vi "Turn to Angle.vi"(3 "PID Gains":T1 {"derivative time (Td, min)" format="%.3f"; "integral time (Ti, min)" format="%.3f"; "proportional gain (Kc)" format="%.3f"}, 4 "Rotation Multiplier":dbl, 5 "Target angle":dbl, 6 "Angle (radians; 0 = right)":dbl) -> (2 "Turn Set Point":dbl)   [LabVIEW 2015]
uses:
  <vilib>/addons/control/pid/pid.llb/PID Control Input Filter (DBL).vi
  <vilib>/addons/control/pid/pid.llb/PID (DBL).vi
  <vilib>/addons/control/pid/NI_PID_pid.lvlib
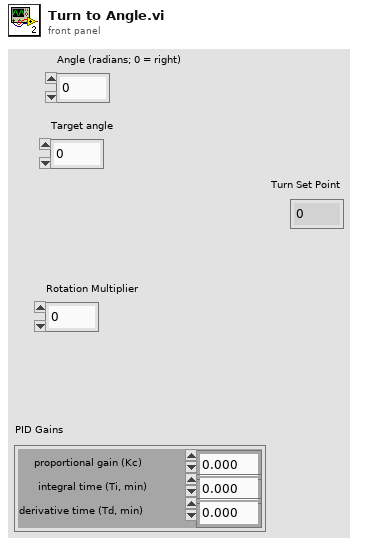
[diagram p1: front panel]
types:
  T1 = cluster{"proportional gain (Kc)":dbl, "integral time (Ti, min)":dbl, "derivative time (Td, min)":dbl}
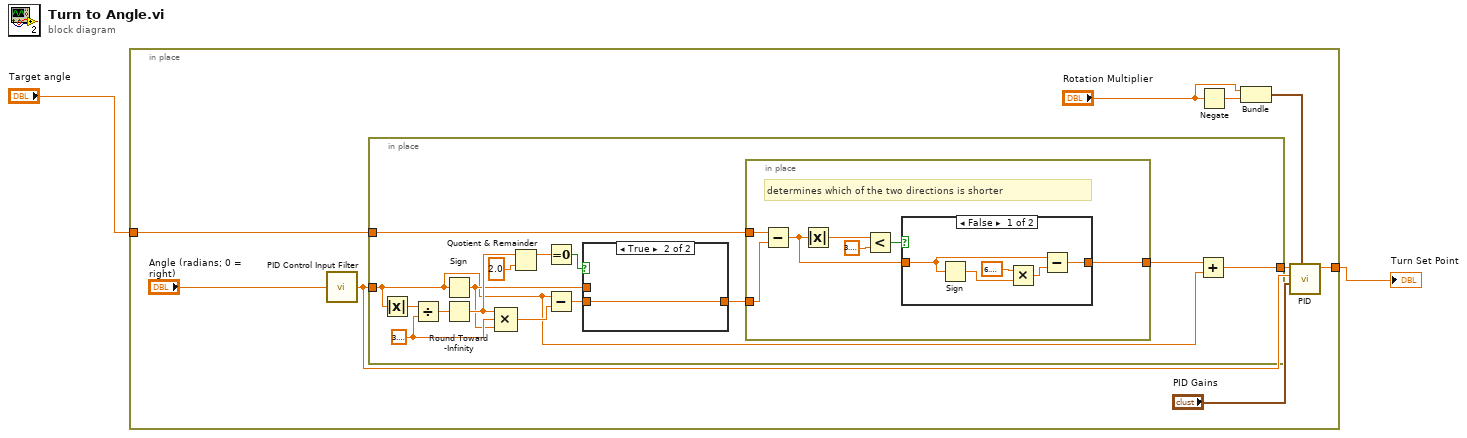
[diagram p0: block diagram]
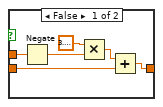
[diagram p3: hidden frame]
diagram:
  n1 = in-place {
    in-place-border: [w11] -> w1
    in-place-border: "Target angle" -> [w5]
    n2 = call-poly <vilib>:"PID Control Input Filter.vi"("input"="Angle (radians; 0 = right)") -> ("output"=w3:dbl)  [unwired: 4 in]
    n3 = in-place {
      in-place-border: w5 -> [w15]
      in-place-border: [w14] -> w4
      in-place-border: w3 -> [w12]
      w23 = 3.141592653589793
      n4 = Absolute Value(x=w12) -> (abs(x)=w26:dbl)
      n5 = Divide(x=w26, y=w23) -> (x/y=w25:dbl)
      n6 = Sign(1:w12) -> (0:w17:dbl)
      n7 = Round Toward -Infinity(1:w25) -> (0:w22:dbl)
      n8 = Compound Arithmetic op=MULTIPLY(w22, w23, w17) -> (w24:dbl)
      n9 = Quotient & Remainder(x=w22, y=2.0) -> (x-y*floor(x/y)=w20:dbl)  [unwired: 1 out]
      n10 = Equal To 0?(x=w20) -> (x = 0?=w18:bool)
      n11 = Subtract(x=w12, y=w24) -> (x-y=w19:dbl)
      n12 = case shown="True" w18 {
        tunnel: [w44 w46] -> w16
        tunnel: w19 -> [w45 w46]
        tunnel: w17 -> [w43 _]
        frame False {
          n13 = Negate(x=w43) -> (-x=w41:dbl)
          n14 = Multiply(x=3.141592653589793, y=w41) -> (x*y=w40:dbl)
          n15 = Add(x=w40, y=w45) -> (x+y=w44:dbl)
        }
        frame True {
        }
      }
      n16 = in-place {
        in-place-border: w15 -> [w28]
        in-place-border: w16 -> [w27]
        in-place-border: [w29] -> w13
        # "determines which of the two directions is shorter"
        n17 = Subtract(x=w28, y=w27) -> (x-y=w33:dbl)
        n18 = Absolute Value(x=w33) -> (abs(x)=w32:dbl)
        n19 = Less?(x=w32, y=3.141592653589793) -> (x < y?=w31:bool)
        n20 = case shown="False" w31 {
          tunnel: w33 -> [w35 w39]
          tunnel: [w34 w39] -> w29
          frame False {
            n21 = Sign(1:w35) -> (0:w37:dbl)
            n22 = Multiply(x=6.283185307179586, y=w37) -> (x*y=w36:dbl)
            n23 = Subtract(x=w35, y=w36) -> (x-y=w34:dbl)
          }
          frame True {
          }
        }
      }
      n24 = Add(x=w13, y=w12) -> (x+y=w14:dbl)
    }
    n25 = Negate(x="Rotation Multiplier") -> (-x=w8:dbl)
    n26 = Bundle("Rotation Multiplier"="Rotation Multiplier", w8) -> (w7:cluster{"Rotation Multiplier":dbl, dbl})  [unwired: 1 in]
    n27 = call-poly <vilib>:"PID.vi"("output range"=w7, "PID gains"="PID Gains", "process variable"=w3, "setpoint"=w4) -> ("output"=w11:dbl)  [unwired: 6 in, 1 out]
  }
  "Turn Set Point" <- w1
